vi "Create Email.vi"   [LabVIEW 2020]
uses:
  Gmail API/Gmail/Gmail.lvclass
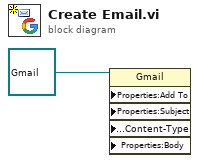
[diagram p0: block diagram]
diagram:
  n1 = property class="Gmail" props=["Properties:Add To", "Properties:Subject", "Properties:Content-Type", "Properties:Body"](reference=refnum<class "Gmail.lvclass"> refnum) -> ()  [unwired: 5 in, 2 out]
